vi "custom stimulus.vi"() -> ()   [LabVIEW 2014]
uses:
  <vilib>/Utility/file.llb/Read From Spreadsheet File (DBL).vi
panel:
  in  "Wait between stimuli (frames)":i32
  in  "Trials Per Power":i32
  in  "Average Power":dbl
  in  "Frames":i32
  in  "Transfer and Run Date Folder After Experiment":bool
  in  "SSH user name":string
  in  "SSH password":string
  in  "Wait before recording (s)":dbl
  in  "Tags":string
  in  "Start Recording":bool
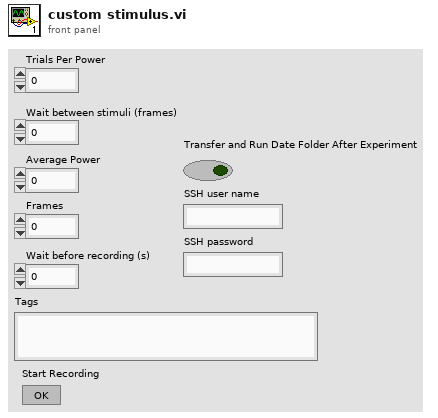
[diagram p1: front panel]
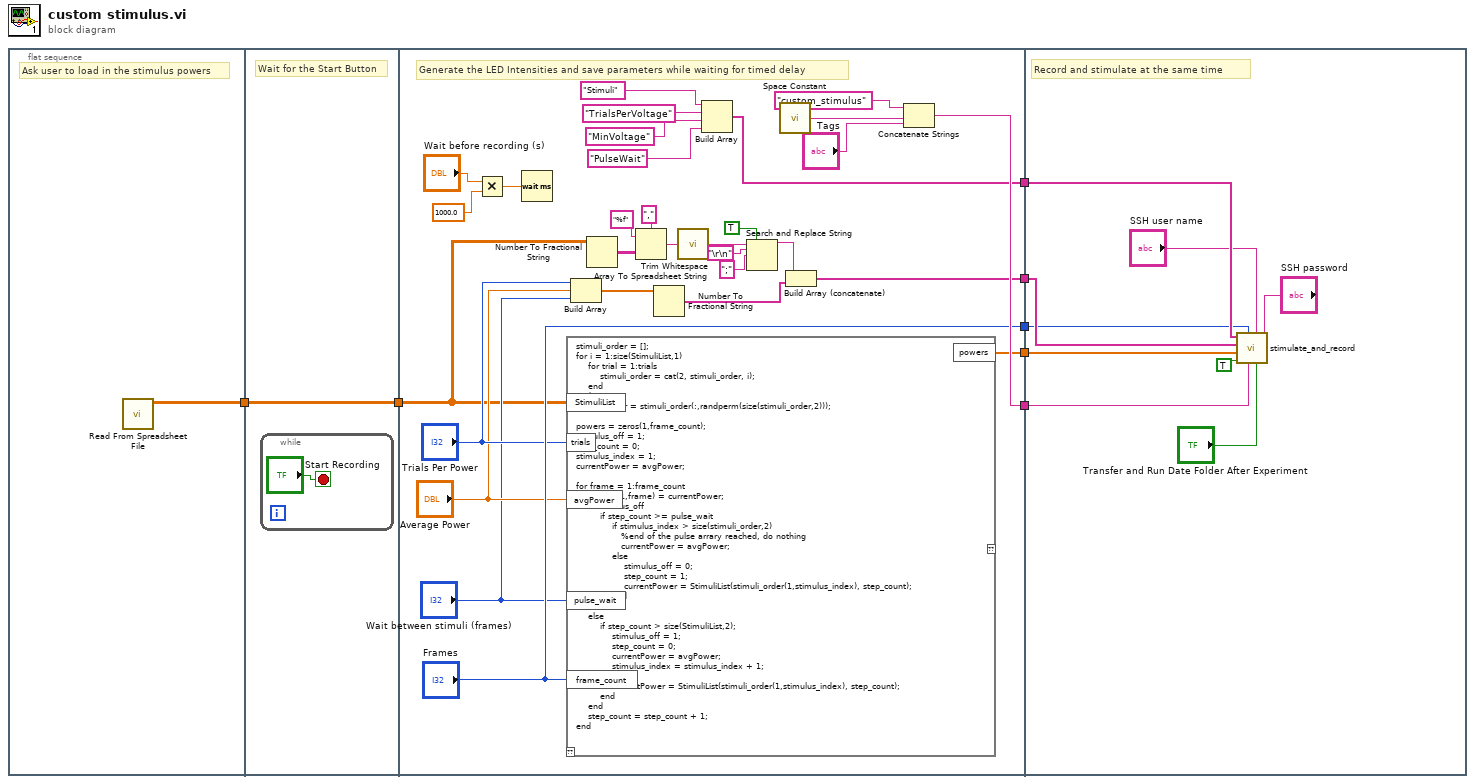
[diagram p0: block diagram]
diagram:
  n1 = flat-sequence {
    tunnel: [w8] -> w3
    tunnel: [w9] -> w4
    tunnel: w3 -> [w9]
    tunnel: [w37] -> w7
    tunnel: [w26] -> w6
    tunnel: [w31] -> w5
    tunnel: w4 -> [w19]
    tunnel: [w25] -> w2
    tunnel: ["Frames"] -> w1
    tunnel: w7 -> [w49]
    tunnel: w6 -> [w47]
    tunnel: w5 -> [w43]
    tunnel: w2 -> [w42]
    tunnel: w1 -> [w41]
    frame #0 {
      # "Ask user to load in the stimulus powers"
      n2 = call-poly <vilib>:"Read From Spreadsheet File.vi"() -> ("all rows"=w8:dbl[][])  [unwired: 7 in, 4 out]
    }
    frame #1 {
      # "Wait for the Start Button"
      n3 = while {
        stop <- "Start Recording" stop-if-true
      }
    }
    frame #2 {
      # "Generate the LED Intensities and save parameters while waiting for timed delay"
      n4 = Multiply(x="Wait before recording (s)", y=1000.0) -> (x*y=w35:dbl)
      n5 = Wait (ms)(milliseconds to wait=w35) -> ()  [unwired: 1 out]
      n6 = script code="stimuli_order = [];\nfor i = 1:size(StimuliList,1)\n    for trial = 1:trials\n        stimuli_order = cat(2, stimuli_order, i);\n    end\nend\nstimuli_order = stimuli_order(:,randperm(size(stimuli_order,2)));\n\npowers = zeros(1,frame_count);\nstimulus_off = 1;\nstep_count = 0;\nstimulus_index = 1;\ncurrentPower = avgPower;\n\nfor frame = 1:frame_count\n    powers(1,frame) = currentPower;\n    if stimulus_off\n        if step_count >= pulse_wait\n            if stimulus_index > size(stimuli_order,2)\n               %end of the pulse arrary reached, do nothing\n               currentPower = avgPower;\n            else\n                stimulus_off = 0;\n                step_count = 1;\n                currentPower = StimuliList(stimuli_order(1,stimulus_index), step_count);\n            end\n        end\n    else\n        if step_count > size(StimuliList,2);\n            stimulus_off = 1;\n            step_count = 0;\n            currentPower = avgPower;\n            stimulus_index = stimulus_index + 1;\n        else\n            currentPower = StimuliList(stimuli_order(1,stimulus_index), step_count);\n        end\n    end\n    step_count = step_count + 1;\nend"("frame_count"="Frames", "trials"="Trials Per Power", "avgPower"="Average Power", "StimuliList"=w19, "pulse_wait"="Wait between stimuli (frames)") -> ("powers"=w25:dbl[])  [unwired: 1 in, 1 out]
      n7 = Build Array("Trials Per Power", "Average Power", "Wait between stimuli (frames)") -> (w20:dbl[])
      n8 = Number To Fractional String(number=w19) -> (F-format string=w18:string[][])  [unwired: 3 in]
      n9 = Array To Spreadsheet String(delimiter (Tab)=",", array=w18, 3:"%f") -> (spreadsheet string=w17:string)
      n10 = Number To Fractional String(number=w20) -> (F-format string=w32:string[])  [unwired: 3 in]
      n11 = call <vilib>:"Trim Whitespace.vi"("string"=w17) -> ("trimmed string"=w16:string)  [unwired: 1 in]
      n12 = Build Array("Stimuli", "TrialsPerVoltage", "MinVoltage", "PulseWait") -> (w26:string[])
      n13 = Search and Replace String(replace all?=TRUE, input string=w16, search string="\r\n", replace string=";") -> (result string=w15:string)  [unwired: 4 in, 3 out]
      n14 = call <vilib>:"Space Constant.vi"() -> ("String"=w39:string)
      n15 = Build Array (concatenate)(w15, w32) -> (w31:string[])
      n16 = Concatenate Strings("custom_stimulus", w39, "Tags") -> (w37:string)
    }
    frame #3 {
      # "Record and stimulate at the same time"
      n17 = call "stimulate_and_record.vi"("SSH password"="SSH password", "Transfer and Run Date Folder After Experiment"="Transfer and Run Date Folder After Experiment", "SSH user name"="SSH user name", "Tags"=w49, "Frames"=w41, "Convert Power to Voltage"=TRUE, "voltages/power"=w42, "parameters"=w43, "parameters headers"=w47) -> ()  [unwired: 3 in]
    }
  }
